vi "example_2_6_f.vi"() -> ()   [LabVIEW 2018]
panel:
  in  "stop":bool
  out "Numeric":dbl format="%.2f"
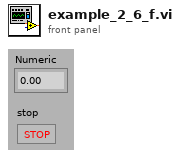
[diagram p1: front panel]
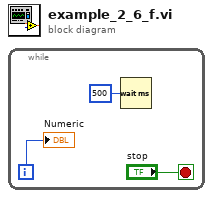
[diagram p0: block diagram]
diagram:
  n1 = while {
    i -> [w2]
    stop <- "stop" stop-if-true
    n2 = Wait (ms)(milliseconds to wait=u32 500) -> ()  [unwired: 1 out]
    "Numeric" <- w2
  }
